vi "Sub_sample_accel_datastream.vi"(11 "Experiment":T1={"Experimental Replay"={"Accelorometer"=array[210000 elements], "Displacement"=array[210000 elements], "dt"=0.0002, "Final Time"=42.0}, "Experimental Results"={"time_average_cycle"=0.0, "measured_frequency"=[], "date_time"="5/2/2024 1:10:00 PM", "estimated_pin_node"=[], "time_cycle_start"=[], "measured_pin_location"=[], "estimated_frequency"=[], "acceleration_data"=[], "accelerometer_sample_rate"=5000.0, "displacement_sample_rate"=5000.0, "time_compare_start"=array[564 elements], "time_subsample_start"=array[564 elements], "time_FEA_start"=array[564 elements], "time_FEA_end"=array[564 elements], "time_cycle_end"=array[564 elements], "time_accelerometer_aquire_start"=array[564 elements], "time_frequency_calculations_start"=array[564 elements], "time_frequency_calculations_end"=array[564 elements], "measured_pin_location_tt"=array[564 elements], "time_ACC_data_collection_start"=80808.5492656, "time_acceleration_data"=array[564 elements], "estimated_pin_location"=array[564 elements], "scaling_factor_Hz_per_pin_to_frequency_resolution"=nan, "Std_Dev_equale_particles_divided_3"=FALSE, "Auto_FFT_length"=FALSE, "windowed_acc_data"=array1x564[564 elements], "FFT"=array1x564[564 elements]}, "FEA Parameters"={"LEMP"={"Eigenvalues"=array[238 elements], "Square Transpose Eigenvectors"=array238x238[56644 elements], "1/deltaStiff"=1e-16}, "nodes of interest"=[19, 20, 21, 22, 23, 24, 25, 26, 27, 28, 29, 30, 31, 32, 33, 34, 35, 36, 37, 38, 39, 40, 41, 42, 43, 44, 45, 46, 47, 48, 49, 50, 51, 52], "all nodes"=[1, 2, 3, 4, 5, 6, 7, 8, 9, 10, 11, 12, 13, 14, 15, 16, 17, 18, 19, 20, 21, 22, 23, 24, 25, 26, 27, 28, 29, 30, 31, 32, 33, 34, 35, 36, 37, 38, 39, 40, 41, 42, 43, 44, 45, 46, 47, 48, 49, 50, 51, 52, 53, 54, 55, 56, 57, 58, 59, 60, 61, 62, 63, 64, 65, 66, 67, 68, 69, 70, 71, 72, 73, 74, 75, 76, 77, 78, 79, 80, 81, 82, 83, 84, 85, 86, 87, 88, 89, 90, 91, 92, 93, 94, 95, 96, 97, 98, 99, 100, 101, 102, 103, 104, 105, 106, 107, 108, 109, 110, 111, 112, 113, 114, 115, 116, 117, 118, 119], "Eigenvalue Method"=enum."0-Local Eigen Modification Procedure", "Mode Count"=3, "initial_pin_node"=0, "Sub Sample"=TRUE}, "Modeling Parameters"={"beam_length"=0.3525, "youngs_modulus"=209500000000.0, "torsion_spring"=0.0, "beam_height"=0.00635, "beam_width"=0.0508, "beam_density"=7900.0, "number_of_FEA_nodes"=120, "FFT_data_length"=4000, "standard_deviation"=2.0, "number_of_particles"=5, "min_FFT_power_value"=0.02, "initial_pin_node"=0, "accelerometer_mass"=0.055, "Max Roller Velocity"=3.32, "Max frequency delta per second"=-320.2269503546099, "Max frequency delta per node"=-1.0, "Min frequency"=49.84843481411623, "Max frequency"=87.165148551616}}) -> (0 "Last pin pos":dbl, 1 "Sample Time":u32, 2 "Displacment sample":dbl[](array[numeric]), 3 "Accelerometer sample":dbl[](array[numeric]), 4 "looping":bool)   [LabVIEW 2021]
panel:
  # "read data from Sub_create_accel_datastream.vi given\n time and desired points"
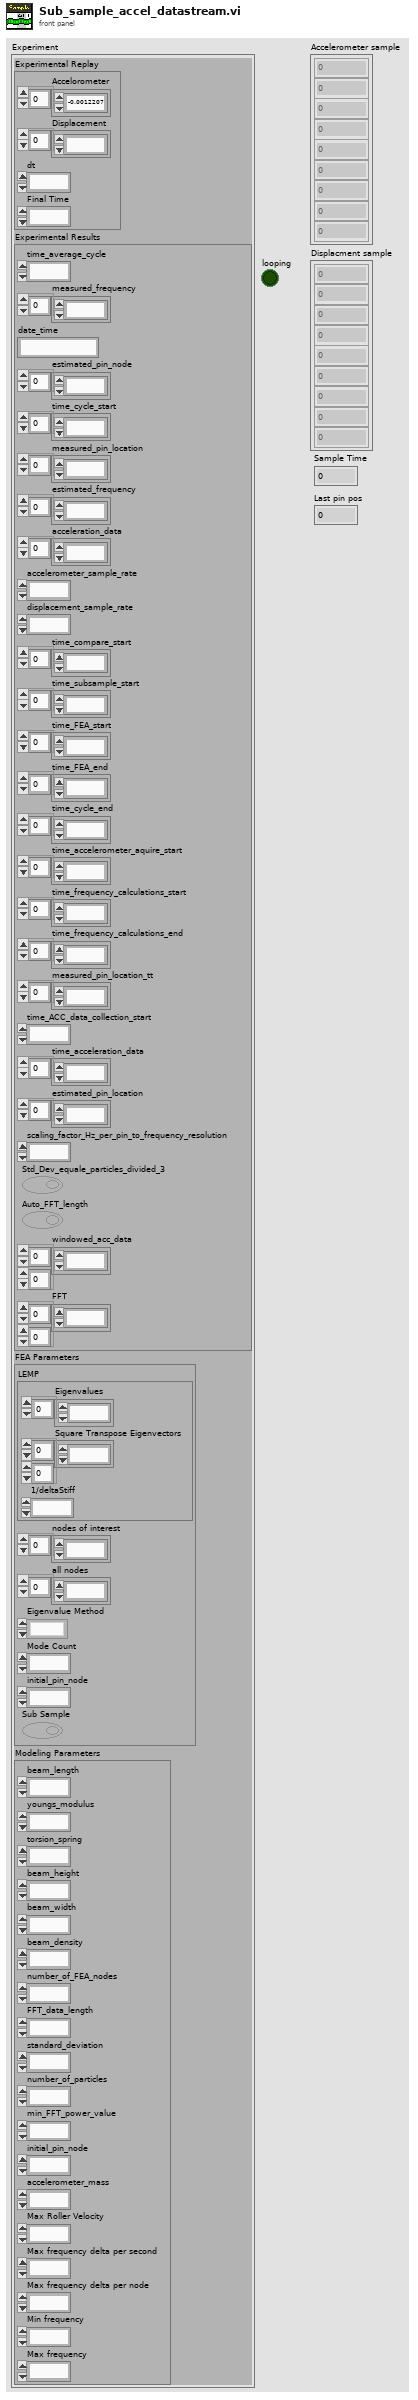
[diagram p1: front panel]
types:
  T1 = cluster{"Experimental Replay":cluster{"Accelorometer":dbl[], "Displacement":dbl[], "dt":dbl, "Final Time":dbl}, "Experimental Results":cluster{"time_average_cycle":dbl, "measured_frequency":dbl[], "date_time":string, "estimated_pin_node":i32[], "time_cycle_start":dbl[], "measured_pin_location":dbl[], "estimated_frequency":dbl[], "acceleration_data":dbl[], "accelerometer_sample_rate":dbl, "displacement_sample_rate":dbl, "time_compare_start":dbl[], "time_subsample_start":dbl[], "time_FEA_start":dbl[], "time_FEA_end":dbl[], "time_cycle_end":dbl[], "time_accelerometer_aquire_start":dbl[], "time_frequency_calculations_start":dbl[], "time_frequency_calculations_end":dbl[], "measured_pin_location_tt":dbl[], "time_ACC_data_collection_start":dbl, "time_acceleration_data":dbl[], "estimated_pin_location":dbl[], "scaling_factor_Hz_per_pin_to_frequency_resolution":dbl, "Std_Dev_equale_particles_divided_3":bool, "Auto_FFT_length":bool, "windowed_acc_data":dbl[][], "FFT":dbl[][]}, "FEA Parameters":cluster{"LEMP":cluster{"Eigenvalues":dbl[], "Square Transpose Eigenvectors":dbl[][], "1/deltaStiff":dbl}, "nodes of interest":i32[], "all nodes":i32[], "Eigenvalue Method":enum16{"0-Local Eigen Modification Procedure", "1-LabVIEW generalized eigenvalues", "2-LabVIEW M^-1K eigenvalues", "3-LabVIEW Cholesky Factorization", "4-Cholesky Factorization CPU SGL", "5-Cholesky Factorization CPU FXP", "6-Cholesky Factorization FPGA SGL", "7-Cholesky Factorization FPGA SGL SCL"}, "Mode Count":i32, "initial_pin_node":i32, "Sub Sample":bool}, "Modeling Parameters":cluster{"beam_length":dbl, "youngs_modulus":dbl, "torsion_spring":dbl, "beam_height":dbl, "beam_width":dbl, "beam_density":dbl, "number_of_FEA_nodes":i32, "FFT_data_length":i32, "standard_deviation":dbl, "number_of_particles":i32, "min_FFT_power_value":dbl, "initial_pin_node":i32, "accelerometer_mass":dbl, "Max Roller Velocity":dbl, "Max frequency delta per second":dbl, "Max frequency delta per node":dbl, "Min frequency":dbl, "Max frequency":dbl}}
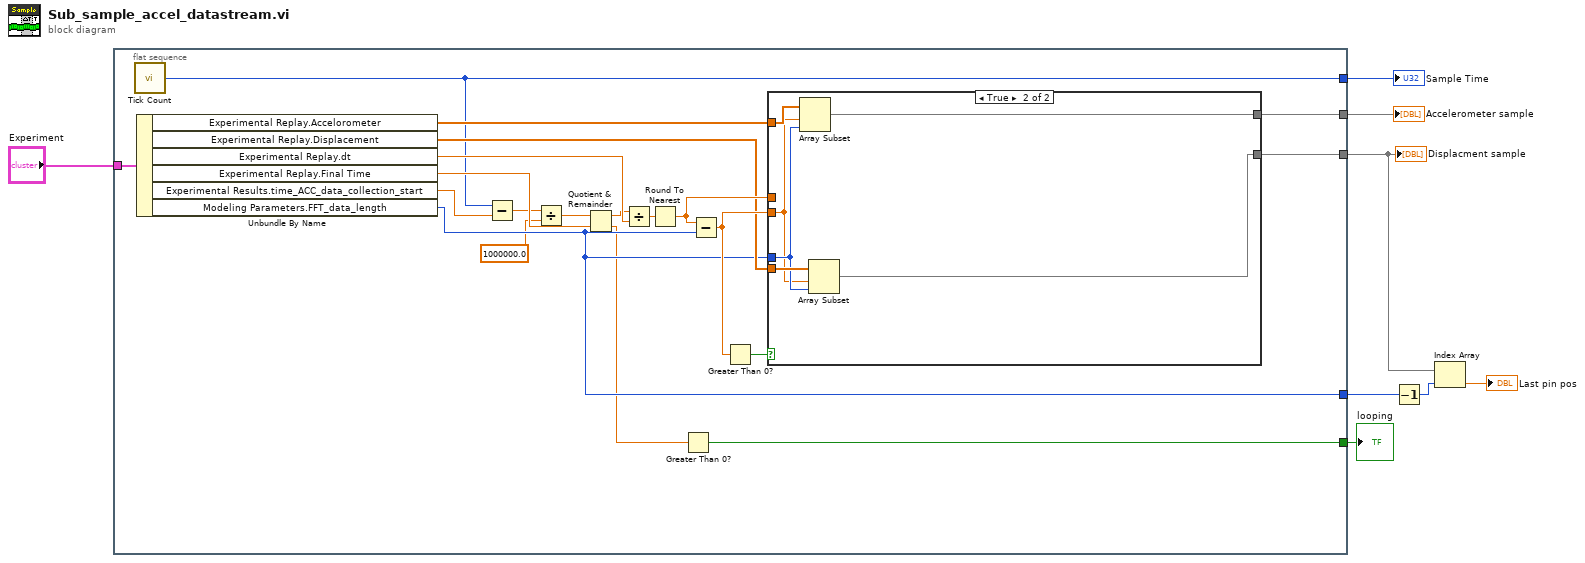
[diagram p0: block diagram]
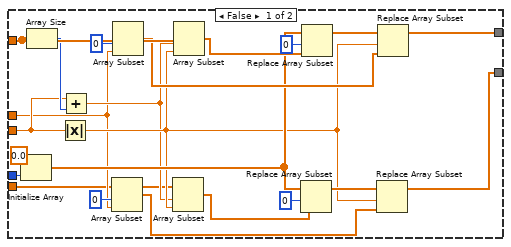
[diagram p2: hidden frame]
diagram:
  n1 = flat-sequence {
    tunnel: "Experiment" -> [w28]
    tunnel: [w25] -> w8
    tunnel: [w21] -> w3
    tunnel: [w16] -> w6
    tunnel: [w15] -> w4
    tunnel: [w13] -> w1
    frame #0 {
      n2 = call "Tick Count"() -> ("Tick Count(uSec)"=w16:u32)
      n3 = Unbundle By Name(w28) -> ("Experimental Replay.Accelorometer"=w26:dbl[], "Experimental Replay.Displacement"=w18:dbl[], "Experimental Replay.dt"=w19:dbl, "Experimental Replay.Final Time"=w20:dbl, "Experimental Results.time_ACC_data_collection_start"=w17:dbl, "Modeling Parameters.FFT_data_length"=w15:i32)
      n4 = Subtract(x=w16, y=w17) -> (x-y=w10:dbl)
      n5 = Divide(x=w10, y=1000000.0) -> (x/y=w11:dbl)
      n6 = Quotient & Remainder(x=w11, y=w20) -> (x-y*floor(x/y)=w14:dbl, floor(x/y)=w12:dbl)
      n7 = Divide(x=w14, y=w19) -> (x/y=w27:dbl)
      n8 = Round To Nearest(number=w27) -> (nearest integer value=w22:dbl)
      n9 = Greater Than 0?(x=w12) -> (x > 0?=w13:bool)
      n10 = Subtract(x=w22, y=w15) -> (x-y=w23:dbl)
      n11 = Greater Than 0?(x=w23) -> (x > 0?=w24:bool)
      n12 = case shown="True" w24 {
        tunnel: w23 -> [w42 w52]
        tunnel: w15 -> [w41 w53]
        tunnel: w26 -> [w50 w56]
        tunnel: [w45 w55] -> w25
        tunnel: w22 -> [w32 _]
        tunnel: [w40 w51] -> w21
        tunnel: w18 -> [w31 w54]
        frame False {
          n13 = Initialize Array(0.0 ("element"), w41) -> (w38:dbl[])
          n14 = Array Size(array=w50) -> (size(s)=w49:i32)
          n15 = Absolute Value(x=w42) -> (abs(x)=w35:dbl)
          n16 = Add(x=w42, y=w49) -> (x+y=w34:dbl)
          n17 = Array Subset(array=w31, index=0, length=w32) -> (w30:dbl[])
          n18 = Array Subset(array=w50, index=0, length=w32) -> (w39:dbl[])
          n19 = Array Subset(array=w31, index=w34, length=w35) -> (w29:dbl[])
          n20 = Array Subset(array=w50, index=w34, length=w35) -> (w44:dbl[])
          n21 = Replace Array Subset(array=w38, new element=w29, index=0) -> (w37:dbl[])
          n22 = Replace Array Subset(array=w38, new element=w44, index=0) -> (w46:dbl[])
          n23 = Replace Array Subset(array=w37, new element=w30, index=w35) -> (w40:dbl[])
          n24 = Replace Array Subset(array=w46, new element=w39, index=w35) -> (w45:dbl[])
        }
        frame True {
          n25 = Array Subset(array=w56, index=w52, length=w53) -> (w55:dbl[])
          n26 = Array Subset(array=w54, index=w52, length=w53) -> (w51:dbl[])
        }
      }
    }
  }
  n27 = Decrement(x=w4) -> (x-1=w5:i32)
  n28 = Index Array(array=w3, index=w5) -> (element=→"Last pin pos":dbl)
  "Accelerometer sample" <- w8
  "Displacment sample" <- w3
  "Sample Time" <- w6
  "looping" <- w1
